vi "Save data.vi"(8 "error in (no error)":errorcluster, 9 "Save data?":bool, 10 "data":waveform(dbl)[](array[waveform]), 11 "file path (dialog if empty)":path) -> (0 "error out":errorcluster)   [LabVIEW 2018]
uses:
  <vilib>/Waveform/WDTOps.llb/WDT Index Channel DBL.vi
  <vilib>/Utility/file.llb/Write Delimited Spreadsheet (DBL).vi
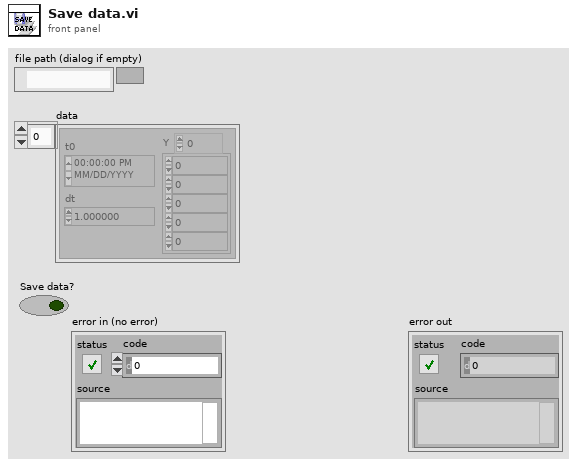
[diagram p1: front panel]
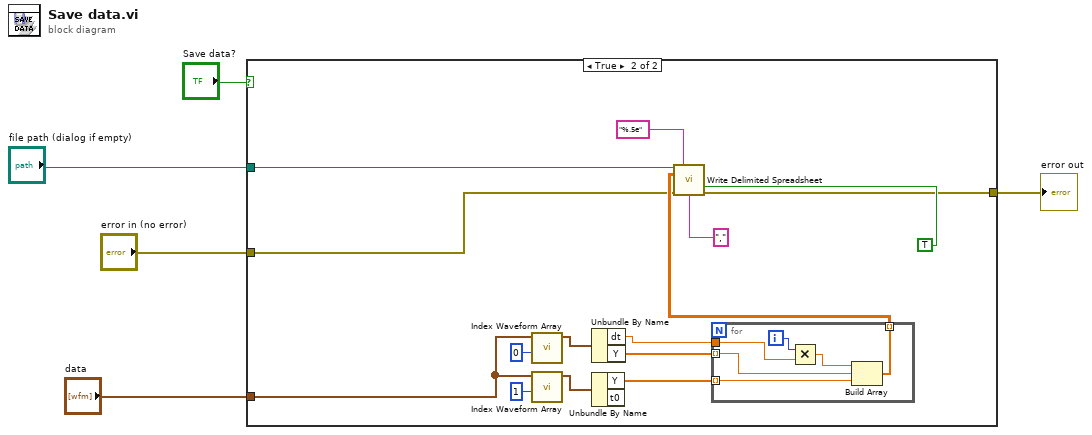
[diagram p0: block diagram]
diagram:
  n1 = case shown="True" "Save data?" {
    tunnel: "data" -> [_ w20]
    tunnel: "file path (dialog if empty)" -> [_ w9]
    tunnel: "error in (no error)" -> [w6 w8]
    tunnel: [w6 w7] -> w1
    frame False {
    }
    frame True {
      n2 = call-poly <vilib>:"Index Waveform Array.vi"("index"=0, "waveform array"=w20) -> ("waveform"=w17:waveform(dbl))  [unwired: 8 in, 1 out]
      n3 = call-poly <vilib>:"Index Waveform Array.vi"("index"=1, "waveform array"=w20) -> ("waveform"=w18:waveform(dbl))  [unwired: 8 in, 1 out]
      n4 = Unbundle By Name(w17) -> ("dt"=w16:dbl, "Y"=w15:dbl[])
      n5 = Unbundle By Name(w18) -> ("Y"=w14:dbl[])  [unwired: 1 out]
      n6 = for {
        tunnel: w16 -> [w26]
        tunnel: w15 -> [w24] mode=indexing
        tunnel: w14 -> [w23] mode=indexing
        tunnel: [w22] -> w13 mode=indexing
        i -> [w27]
        n7 = Multiply(x=w27, y=w26) -> (x*y=w25:dbl)
        n8 = Build Array(w25, w24, w23) -> (w22:dbl[])
      }
      n9 = call-poly <vilib>:"Write Delimited Spreadsheet.vi"("file path (dialog if empty)"=w9, "format (%.3f)"="%.5e", "2D data"=w13, "append to file? (new file:F)"=TRUE, "error in (no error)"=w8, "delimiter (\\t)"="," ("delimiter (Tab)")) -> ("error out"=w7:errorcluster)  [unwired: 8 in, 1 out]
    }
  }
  "error out" <- w1
